vi "AlliGator Phasor Harmonic Storage [SGL].vi"(8 "Error In":errorcluster, 9 "Current Phasor Harmonic":T2 {"Base Frequency" min=0.0 max=255000000.0}, 10 "Default Name (\"Phasor Harmonic\")":string="Phasor Harmonic", 11 "Action":T1=enum."Store Multiple Harmonics") -> (0 "Error Out":errorcluster, 1 "Current Phasor Harmonic":T2 {"Base Frequency" min=0.0 max=255000000.0}, 2 "Current Phasor Harmonic Name":string, 3 "Current Phasor Harmonic Index":i32, 4 "Old Phasor Harmonic Name":string, 5 "Message":string)   [LabVIEW 2021, in "AlliGator Phasor Harmonics.lvlib"]
uses:
  AlliGator Phasor Harmonics.lvlib
  Phasor/Phasor Harmonic Data.ctl
  Phasor Plot/AlliGator Phasor Harmonic Manager Actions.ctl
  Globals, Variables, Constants/AlliGator Variables List.ctl
  Variant/Variant to Data/Variant to [I32].vi
  Globals, Variables, Constants/AlliGator Globals, Variables & Constants.lvlib
  Variant/Variant to Data/Variant to Data.lvlib
  Phasor Plot/AlliGator Phasor Plot.lvlib
  Phasor/Phasor.lvlib
  Strings/Strings.lvlib
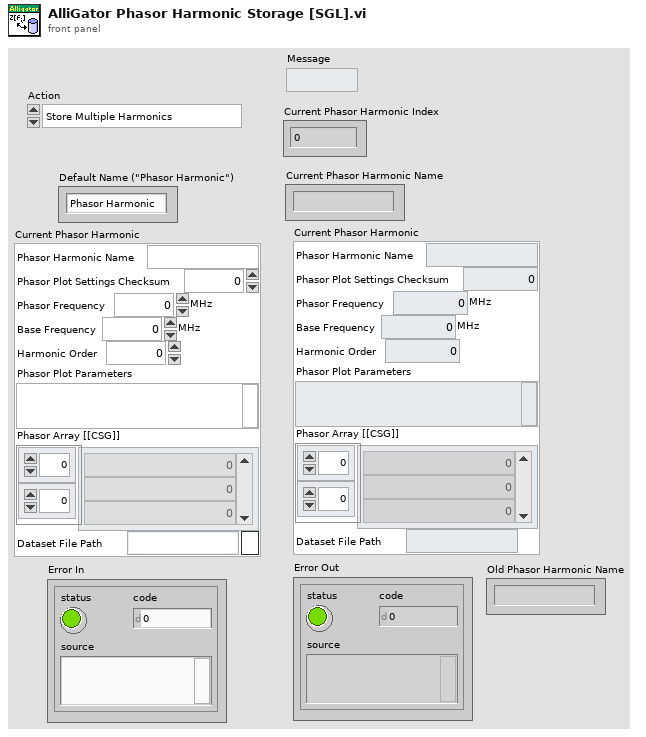
[diagram p1: front panel]
types:
  T1 = typedef "AlliGator Phasor Plot.lvlib/AlliGator Phasor Harmonic Manager Actions.ctl" = enum16{"Undefined", "Delete Current Harmonic", "Delete Multiple Harmonics", "Delete All Harmonics", "Swap Harmonics", "Insert Harmonics", "Rename Current Harmonic", "Store New Harmonic", "Store Multiple Harmonics", "Select Next Harmonic", "Select Previous Harmonic", "Update Phasor Harmonic Manager Window"}
  T2 = typedef "Phasor.lvlib/Phasor Harmonic Data.ctl" = cluster{"Phasor Harmonic Name":string, "Phasor Plot Settings Checksum":u64, "Phasor Frequency":dbl[unit], "Base Frequency":dbl[unit], "Harmonic Order":u8, "Phasor Plot Parameters":string, "Phasor Array [[CSG]]":csg[][], "Dataset File Path":path}
  T3 = typedef "AlliGator Globals, Variables & Constants.lvlib/AlliGator Variables List.ctl" = enum16{"---- GUI ----", "GUI:Initialization Status", "GUI:State Indicators Refnum", "GUI:Original AlliGator Menu Items", "GUI:Current Action Loop State", "GUI:Script in progress", "GUI:Playback", "GUI:Loop Playback", "GUI:Search ROI Used", "GUI:Search ROI", "Decay Graph Max Legend Size", "Intensity Graph Max Legend Size", "Decay Statistics Graph Max Legend Size", "Phasor Graph Max Legend Size", "Phasor Ratio Graph Max Legend Size", "Lifetime Graph Max Legend Size", "---- Files ----", "Files:Export Dataset Frames as Individual Files", "Files:Show Batch Export Help Balloons", "Files:Frames in Dataset", "Files:ptu File Frame Start Indices", "Files:Current Frame in Dataset", "Files:Current Frame Timestamp", "Files:Dataset Loaded", "Files:Dataset Metadata", "Files:Dataset Channel", "Files:Dataset Data Description", "Files:Background Dataset Metadata", "Files:Background Dataset Channel", "Files:Background Dataset Data Description", "Files:Background File Subtraction", "Files:Background File Path", "Files:Background File Pile-up Correction", "Files:Background File Pixel Well Capacity", "Files:Background File Scaling Factor", "Files:Current Dataset Load Settings", "Files:Dataset Path", "Files:ICCD-specific Information", "Files:Macrotime Gate Separation", "------ Python Plugins ------", "Python Plugins:Information", "Python Plugins:Python Session", "Python Plugins:Valid Python Session?", "---- Source Image ----", "Source Image:ROIs", "Source Image:Current ROI", "Source Image:ROI Event Refnum", "X_Source Image:Display Range", "X_Source Image:Palette Information", "X_Source Image:Type of Displayed Image", "X_Time Gate Slider", "Source Image:Palette List", "Source Image:Scale", "Source Image:ROI Overlay Color", "Source Image:Overlay to Erase", "Source Image:Is Displayed Image Accumulated", "Source Image:White Light Image Modified", "Source Image:Mask Image Modified", "---- Image Profile Window ----", "Image Profile:Window Event Refnum", "Image Profile:IntensityType", "Image Profile:Intensity Average Type", "Image Profile:Intensity-weighted SDV", "Image Profile:Box Profile Type", "Image Profile:Window Open", "Image Profile:Plotted Fit Parameter", "------ Phasor Graph -------", "Phasor Graph:Show Line", "---- Phasor Plot ---", "Phasor Plot:Parameters Changed", "Phasor Plot:FLI Dataset Modified since last Calculation", "Phasor Harmonics Data", "Selected Phasor Harmonics", "Phasor Harmonic Manager Event Refnum", "Phasor Plot:ROIs", "Phasor Plot:Current ROI", "Phasor Plot:ROI Event Refnum", "Phasor Plot:Image Reference Points", "Phasor Plot:Computed", "Phasor Plot:Palette Information", "Phasor Plot:Palette List", "Phasor Plot:Phasor Ratio Palette Information", "Phasor Plot:Phasor Ratio Palette List", "Phasor Plot:Image Scale", "Phasor Plot:Image Overlay to Erase", "Phasor Plot:Image Elements to Update", "Phasor Plot:Current Calculation Parameters", "Phasor Plot:Current Calibration Options", "Phasor Plot:Reset Cumulated Phasor Plot", "Phasor Plot:Reference 1", "Phasor Plot:Lifetime Reference 1", "Phasor Plot:Reference 1 Frequency", "Phasor Plot:Reference 2", "Phasor Plot:Lifetime Reference 2", "Phasor Plot:Reference 2 Frequency", "---- Decay Analysis ----", "Number of Selected Decays to Fit", "LS Fit Results", "LAR Fit Results", "BS Fit Results", "Last Decay Max - Min", "Best Fit Parameters", "Best Fit Parameter Names", "Actual Size X", "Actual Size Y", "Binning X", "Binning Y", "Actual # Gates", "Dataset Number", "Gates to...", "Gates Skipped", "Gates to keep", "Gate Step", "Gate Separation", "Reversed Gates", "Pile-up Correction", "Pixel Well Capacity", "Background Subtracted", "Background Subtraction Method", "Background Definition Range", "Background File (deprecated)", "Number of Dataset Accumulated", "Array of Accumulated Dataset Paths", "Do Averaged Datasets", "Destination File Path", "Process Plot Target", "Use 1/D as Phasor Frequency", "---- Decay Fit Parameter Map -----", "Decay Fit Parameter Map:Palette Information", "Decay Fit Parameter Map:Palette List", "Decay Fit Parameter Map:X Resolution", "Decay Fit Parameter Map:Y Resolution", "---- Parameter Map ----", "Parameter Map:Palette Information", "Parameter Map:Palette List", "------- Local Decay Window ---------", "Local Decay Graph Window:Event Refnum", "Local Decay Graph Window:Use normalized IRF for convolution", "----- Miscellaneous ----", "Misc:Skippable Dialog Windows Status"}
  T4 = typedef "AlliGator Phasor Plot.lvlib/AlliGator Phasor Harmonic Manager Event Refnum.ctl" = refnum<user-event>
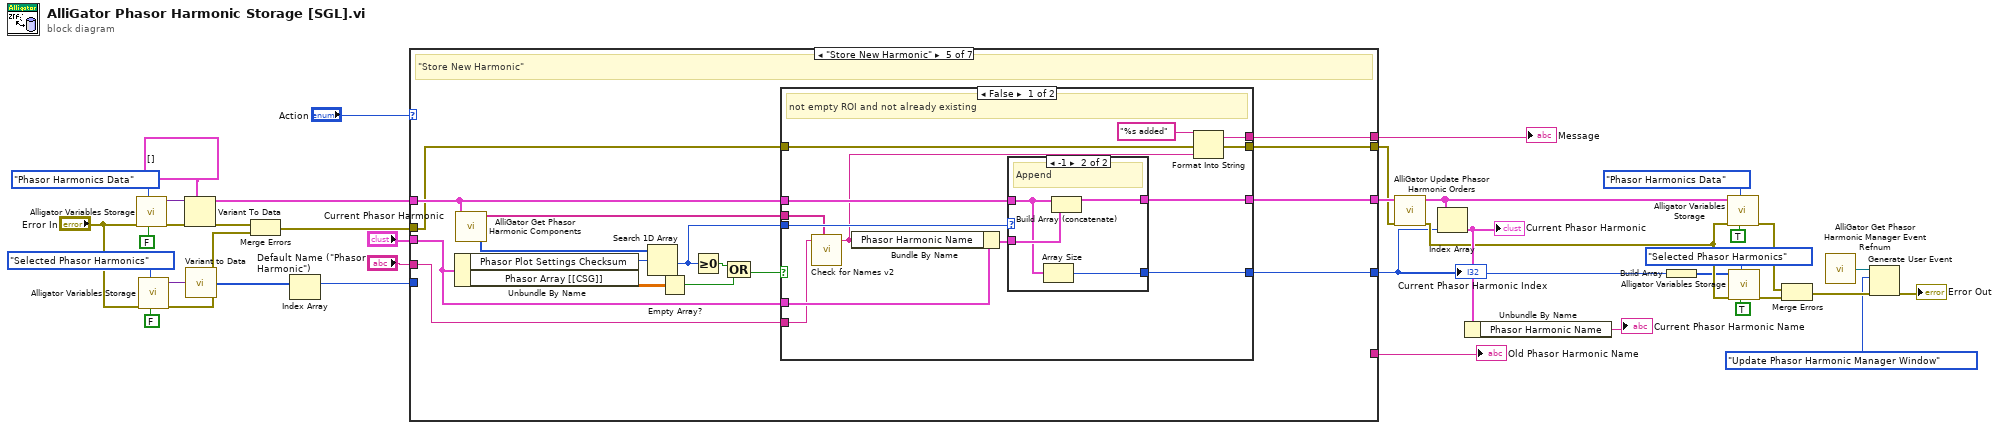
[diagram p0: block diagram]
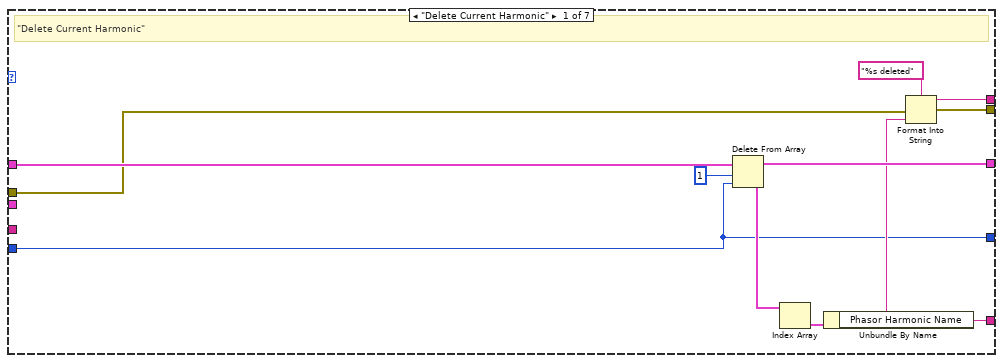
[diagram p2: hidden frame]
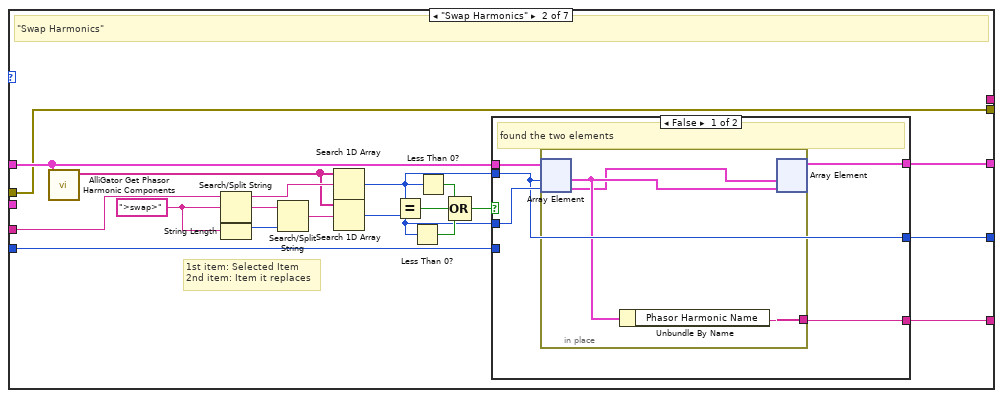
[diagram p3: hidden frame]
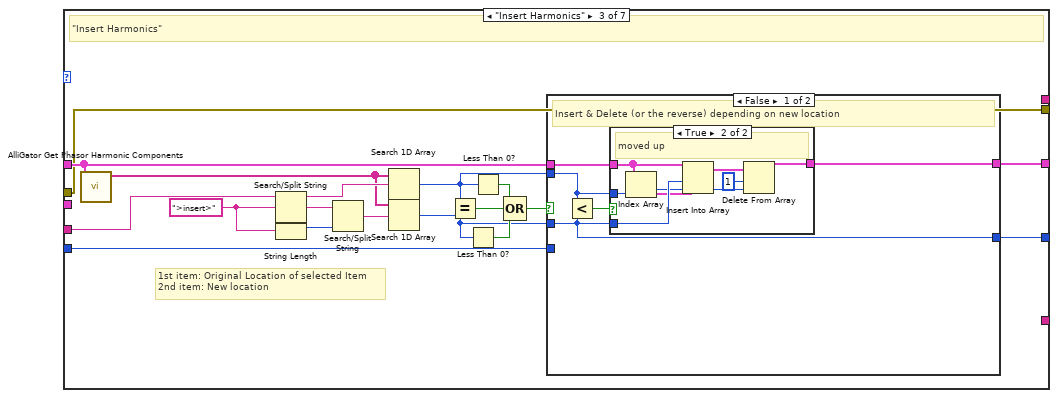
[diagram p5: hidden frame]
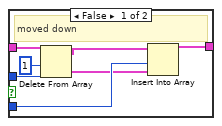
[diagram p6: hidden frame]
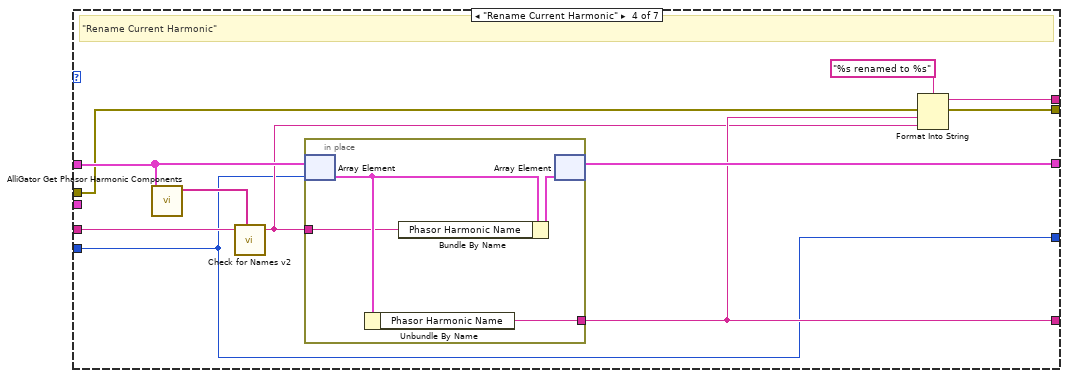
[diagram p8: hidden frame]
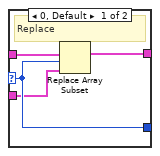
[diagram p9: hidden frame]
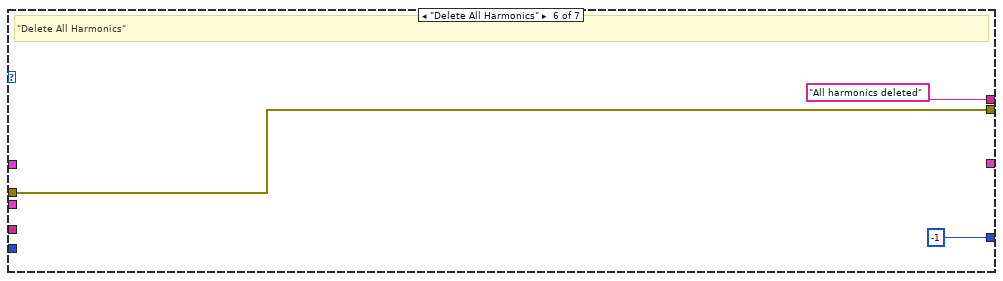
[diagram p11: hidden frame]
diagram:
  n1 = call "Alligator Variables Storage.vi"("Get(F)/Set"=FALSE, "AlliGator Variable"=AlliGator_Variables_List."Phasor Harmonics Data" ("Alligator Variable"), "Error In"="Error In") -> ("Error Out"=w36:errorcluster, "Data out"=w37:variant)  [unwired: 6 in, 1 out]
  n2 = call "Alligator Variables Storage.vi"("Get(F)/Set"=FALSE, "AlliGator Variable"=AlliGator_Variables_List."Selected Phasor Harmonics" ("Alligator Variable"), "Error In"="Error In") -> ("Error Out"=w26:errorcluster, "Data out"=w31:variant)  [unwired: 6 in, 1 out]
  n3 = Variant To Data(error in=w36, type=T2[] [] ("Stored ROIs in"), Variant=w37) -> (data=w19:T2[], error out=w25:errorcluster)
  n4 = call-poly "Variant to Data.vi"("Variant"=w31) -> ("Value"=w18:i32[])  [unwired: 8 in]
  n5 = Merge Errors(w25, w26) -> (w6:errorcluster)
  n6 = Index Array(array=w18) -> (element=w2:i32)  [unwired: 1 in]
  n7 = case shown="\"Store New Harmonic\"" "Action" {
    tunnel: w19 -> [w49 w52 w80 w128 w144 _ w177]
    tunnel: w2 -> [w39 w68 w96 w118 _ _ _]
    tunnel: [w47 w67 w95 w127 w148 _ w177] -> w11
    tunnel: [w39 w66 w94 w118 w147 -1 ("index of element") _] -> w1
    tunnel: "Current Phasor Harmonic" -> [_ _ _ _ w136 _ _]
    tunnel: "Default Name (\"Phasor Harmonic\")" -> [_ w64 w93 w126 w146 _ _]
    tunnel: [w41 w65 _ w122 _ _ _] -> w15
    tunnel: w6 -> [w40 w50 w79 w125 w135 w174 w176]
    tunnel: [w42 w50 w79 w124 w133 w174 w176] -> w5
    tunnel: [w43 _ _ w123 w134 "All harmonics deleted" ("format string") _] -> w4
    frame "Delete Current Harmonic" {
      # "\"Delete Current Harmonic\""
      n8 = Delete From Array(array=w49, length=1, index=w39) -> (deleted portion=w46:T2[], array with subset deleted=w47:T2[])
      n9 = Index Array(array=w46) -> (element=w45:T2)  [unwired: 1 in]
      n10 = Unbundle By Name(w45) -> ("Phasor Harmonic Name"=w41:string)
      n11 = Format Into String(format string="%s deleted", error in=w40, w41) -> (resulting string=w43:string, error out=w42:errorcluster)  [unwired: 1 in]
    }
    frame "Swap Harmonics" {
      w62 = ">swap>" ("search string/char (-)")
      # "1st item: Selected Item\n2nd item: Item it replaces"
      # "\"Swap Harmonics\""
      n12 = call "AlliGator Get Phasor Harmonic Components.vi"("Stored Phasor Harmonics"=w52) -> ("Phasor Harmonic Names"=w51:string[])  [unwired: 4 in, 6 out]
      n13 = Search/Split String(string=w64, search string/char (-)=w62) -> (substring before match=w60:string, match + rest of string=w63:string)  [unwired: 1 in, 1 out]
      n14 = String Length(string=w62) -> (length=w61:i32)
      n15 = Search/Split String(string=w63, offset (0)=w61) -> (match + rest of string=w59:string)  [unwired: 1 in, 2 out]
      n16 = Search 1D Array(1D array=w51, element=w60) -> (index of element=w54:i32)  [unwired: 1 in]
      n17 = Search 1D Array(1D array=w51, element=w59) -> (index of element=w53:i32)  [unwired: 1 in]
      n18 = Equal?(x=w54, y=w53) -> (x = y?=w56:bool)
      n19 = Less Than 0?(x=w53) -> (x < 0?=w57:bool)
      n20 = Less Than 0?(x=w54) -> (x < 0?=w58:bool)
      n21 = Compound Arithmetic op=OR(w58, w56, w57) -> (w55:bool)
      n22 = case shown="False" w55 {
        tunnel: w68 -> [_ w77]
        tunnel: [w72 w78] -> w67
        tunnel: [w69 w77] -> w66
        tunnel: [w70 _] -> w65
        tunnel: w52 -> [w73 w78]
        tunnel: w54 -> [w69 _]
        tunnel: w53 -> [w71 _]
        frame False {
          # "found the two elements"
          n23 = in-place {
            in-place-border: [w76] -> w70
            n24 = in-place-array #1(w73, w69, w71) -> (w75:T2, w74:T2)
            n25 = Unbundle By Name(w75) -> ("Phasor Harmonic Name"=w76:string)
            n26 = in-place-array #1(w74, w75) -> (w72:T2[])  [unwired: 2 out]
          }
        }
        frame True {
          # "no action"
        }
      }
    }
    frame "Insert Harmonics" {
      w91 = ">insert>" ("search string/char (-)")
      # "1st item: Original Location of selected Item\n2nd item: New location"
      # "\"Insert Harmonics\""
      n27 = call "AlliGator Get Phasor Harmonic Components.vi"("Stored Phasor Harmonics"=w80) -> ("Phasor Harmonic Names"=w88:string[])  [unwired: 4 in, 6 out]
      n28 = Search/Split String(string=w93, search string/char (-)=w91) -> (substring before match=w89:string, match + rest of string=w92:string)  [unwired: 1 in, 1 out]
      n29 = String Length(string=w91) -> (length=w90:i32)
      n30 = Search/Split String(string=w92, offset (0)=w90) -> (match + rest of string=w87:string)  [unwired: 1 in, 2 out]
      n31 = Search 1D Array(1D array=w88, element=w89) -> (index of element=w82:i32)  [unwired: 1 in]
      n32 = Search 1D Array(1D array=w88, element=w87) -> (index of element=w81:i32)  [unwired: 1 in]
      n33 = Equal?(x=w82, y=w81) -> (x = y?=w84:bool)
      n34 = Less Than 0?(x=w81) -> (x < 0?=w85:bool)
      n35 = Less Than 0?(x=w82) -> (x < 0?=w86:bool)
      n36 = Compound Arithmetic op=OR(w86, w84, w85) -> (w83:bool)
      n37 = case shown="False" w83 {
        tunnel: w96 -> [_ w116]
        tunnel: [w98 w117] -> w95
        tunnel: [w97 w116] -> w94
        tunnel: w80 -> [w100 w117]
        tunnel: w82 -> [w99 _]
        tunnel: w81 -> [w97 _]
        frame False {
          # "Insert & Delete (or the reverse) depending on new location"
          n38 = Less?(x=w99, y=w97) -> (x < y?=w101:bool)
          n39 = case shown="True" w101 {
            tunnel: w100 -> [w108 w115]
            tunnel: w99 -> [w107 w111]
            tunnel: w97 -> [w103 w114]
            tunnel: [w104 w109] -> w98
            frame False {
              # "moved down"
              n40 = Delete From Array(array=w108, length=1, index=w107) -> (deleted portion=w102:T2[], array with subset deleted=w105:T2[])
              n41 = Insert Into Array(array=w105, index=w103, new element=w102) -> (w104:T2[])
            }
            frame True {
              # "moved up"
              n42 = Index Array(array=w115, index=w111) -> (element=w113:T2)
              n43 = Insert Into Array(array=w115, index=w114, new element=w113) -> (w112:T2[])
              n44 = Delete From Array(array=w112, length=1, index=w111) -> (array with subset deleted=w109:T2[])  [unwired: 1 out]
            }
          }
        }
        frame True {
          # "no action"
        }
      }
    }
    frame "Rename Current Harmonic" {
      # "\"Rename Current Harmonic\""
      n45 = call "AlliGator Get Phasor Harmonic Components.vi"("Stored Phasor Harmonics"=w128) -> ("Phasor Harmonic Names"=w121:string[])  [unwired: 4 in, 6 out]
      n46 = call "Check for Names v2.vi"("New Name"=w126, "Name List"=w121) -> ("New Name"=w119:string)  [unwired: 4 in, 3 out]
      n47 = in-place {
        in-place-border: w119 -> [w129]
        in-place-border: [w130] -> w122
        n48 = in-place-array #2(w128, w118) -> (w131:T2)
        n49 = Unbundle By Name(w131) -> ("Phasor Harmonic Name"=w130:string)
        n50 = Bundle By Name(cluster=w131, "Phasor Harmonic Name"=w129) -> (w132:T2)
        n51 = in-place-array #2(w132) -> (w127:T2[])  [unwired: 1 out]
      }
      n52 = Format Into String(format string="%s renamed to %s", error in=w125, w122, w119) -> (resulting string=w123:string, error out=w124:errorcluster)  [unwired: 1 in]
    }
    frame "Store New Harmonic" {
      # "\"Store New Harmonic\""
      n53 = Unbundle By Name(w136) -> ("Phasor Plot Settings Checksum"=w142:u64, "Phasor Array [[CSG]]"=w140:csg[][])
      n54 = call "AlliGator Get Phasor Harmonic Components.vi"("Stored Phasor Harmonics"=w144) -> ("Phasor Harmonic Names"=w143:string[], "Phasor Harmonic Checksums"=w145:u64[])  [unwired: 4 in, 5 out]
      n55 = Search 1D Array(1D array=w145, element=w142) -> (index of element=w137:i32)  [unwired: 1 in]
      n56 = Empty Array?(array=w140) -> (empty?=w139:bool)
      n57 = Greater Or Equal To 0?(x=w137) -> (x >= 0?=w141:bool)
      n58 = Compound Arithmetic op=OR(w141, w139) -> (w138:bool)
      n59 = case shown="False" w138 {
        tunnel: [w161 w172] -> w148
        tunnel: [w160 w171] -> w147
        tunnel: w144 -> [w159 w172]
        tunnel: w146 -> [w156 _]
        tunnel: w143 -> [w155 _]
        tunnel: w137 -> [w157 w171]
        tunnel: w136 -> [w158 _]
        tunnel: w135 -> [w151 w170]
        tunnel: [w150 _] -> w134
        tunnel: [w149 w170] -> w133
        frame False {
          # "not empty ROI and not already existing"
          n60 = call "Check for Names v2.vi"("New Name"=w156, "Name List"=w155) -> ("New Name"=w153:string)  [unwired: 4 in, 3 out]
          n61 = Bundle By Name(cluster=w158, "Phasor Harmonic Name"=w153) -> (w154:T2)
          n62 = case shown="-1" w157 {
            selector: w157 -> [w164 _]
            tunnel: [w163 w169] -> w161
            tunnel: [w164 w168] -> w160
            tunnel: w154 -> [w162 w167]
            tunnel: w159 -> [w165 w166]
            frame 0, Default {
              # "Replace"
              n63 = Replace Array Subset(array=w165, new element=w162, index=w164) -> (w163:T2[])
            }
            frame -1 {
              # "Append"
              n64 = Array Size(array=w166) -> (size(s)=w168:i32)
              n65 = Build Array (concatenate)(w166, w167) -> (w169:T2[])
            }
          }
          n66 = Format Into String(format string="%s added", error in=w151, w153) -> (resulting string=w150:string, error out=w149:errorcluster)  [unwired: 1 in]
        }
        frame True {
          # "no need to change or empty ROI"
        }
      }
    }
    frame "Delete All Harmonics" {
      # "\"Delete All Harmonics\""
    }
    frame Default {
    }
  }
  "Current Phasor Harmonic Index" <- w1
  "Old Phasor Harmonic Name" <- w15
  "Message" <- w4
  n67 = call "AlliGator Update Phasor Harmonic Orders.vi"("Error In"=w5, "Stored Phasor Harmonics in"=w11) -> ("Error Out"=w7:errorcluster, "Stored Phasor Harmonics out"=w8:T2[])  [unwired: 8 in]
  n68 = Index Array(array=w8, index=w1) -> (element=w10:T2)
  "Current Phasor Harmonic" <- w10
  n69 = Unbundle By Name(w10) -> ("Phasor Harmonic Name"=→"Current Phasor Harmonic Name":string)
  n70 = Build Array(w1) -> (w3:i32[])
  n71 = call "Alligator Variables Storage.vi"("Get(F)/Set"=TRUE, "AlliGator Variable"=AlliGator_Variables_List."Phasor Harmonics Data" ("Alligator Variable"), "Error In"=w7, "Data in"=w8) -> ("Error Out"=w23:errorcluster)  [unwired: 5 in, 2 out]
  n72 = call "Alligator Variables Storage.vi"("Get(F)/Set"=TRUE, "AlliGator Variable"=AlliGator_Variables_List."Selected Phasor Harmonics" ("Alligator Variable"), "Error In"=w7, "Data in"=w3) -> ("Error Out"=w24:errorcluster)  [unwired: 5 in, 2 out]
  n73 = Merge Errors(w23, w24) -> (w21:errorcluster)
  n74 = call "AlliGator Get Phasor Harmonic Manager Event Refnum.vi"() -> ("Phasor Harmonic Manager Event Refnum"=w13:T4)
  n75 = Generate User Event(user event=w13, event data cluster=AlliGator_Phasor_Harmonic_Manager_Actions."Update Phasor Harmonic Manager Window" ("event data"), error in=w21) -> (error out=→"Error Out":errorcluster)  [unwired: 1 in, 1 out]
